vi "UNIT_TEST_INTAKE.vi"() -> ()   [LabVIEW 2019]
uses:
  <vilib>/Rock Robotics/WPI/Solenoid/WPI_SolenoidValue.ctl
panel:
  out "Hopper Output 2":T1=enum."Reverse"
  out "Intake Output 2":T1=enum."Reverse"
  in  "Hopper Input 2":T1=enum."Reverse"
  in  "Intake Input 2":T1=enum."Reverse"
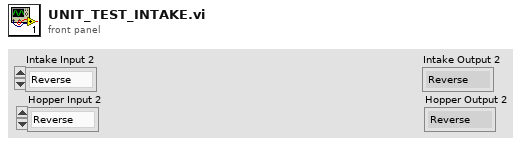
[diagram p1: front panel]
types:
  T1 = typedef "WPI_SolenoidValue.ctl" = enum16{"Off", "On", "Forward", "Reverse"}
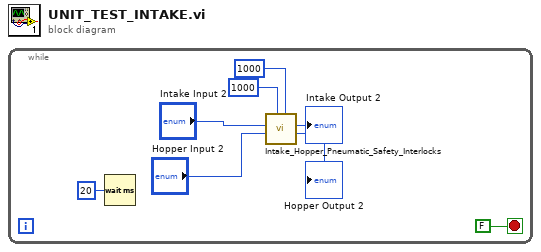
[diagram p0: block diagram]
diagram:
  n1 = while {
    stop <- FALSE stop-if-true
    n2 = Wait (ms)(milliseconds to wait=u32 20) -> ()  [unwired: 1 out]
    n3 = call "Intake_Hopper_Pneumatic_Safety_Interlocks.vi"("retract delay(ms)"=u32 1000, "extend delay(ms)"=u32 1000, "Hopper Input"="Hopper Input 2", "Intake Input"="Intake Input 2") -> ("Hopper Output"=→"Hopper Output 2":T1, "Intake Output"=→"Intake Output 2":T1)  [unwired: 6 in]
  }
